vi "Programer.vi"(7 "ID":T1, 8 "error in":errorcluster, 9 "version path":path=path "C:/4.9.12.6034", 10 "Boolean refs":refnum<vi>[](array[refnum]), 11 "Commands":string[](array[string])) -> (0 "error out":errorcluster, 1 "error?":bool, 2 "Checksum":string, 3 "Response":string)   [LabVIEW 2021]
uses:
  controls/ID.ctl
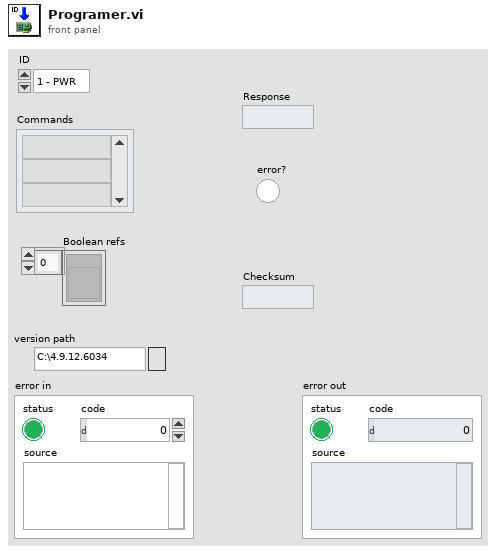
[diagram p1: front panel]
types:
  T1 = typedef "ID.ctl" = enum16{"1 - PWR", "2 - SM", "3 - DC", "4 - DM", "5 - WS", "6 - DS", "7 - WC", "8 - WA", "9 - WM", "10 - DA", "11 - WH", "12 - DH"}
  T2 = cluster{"accent s color":u32, "accent s color":u32}
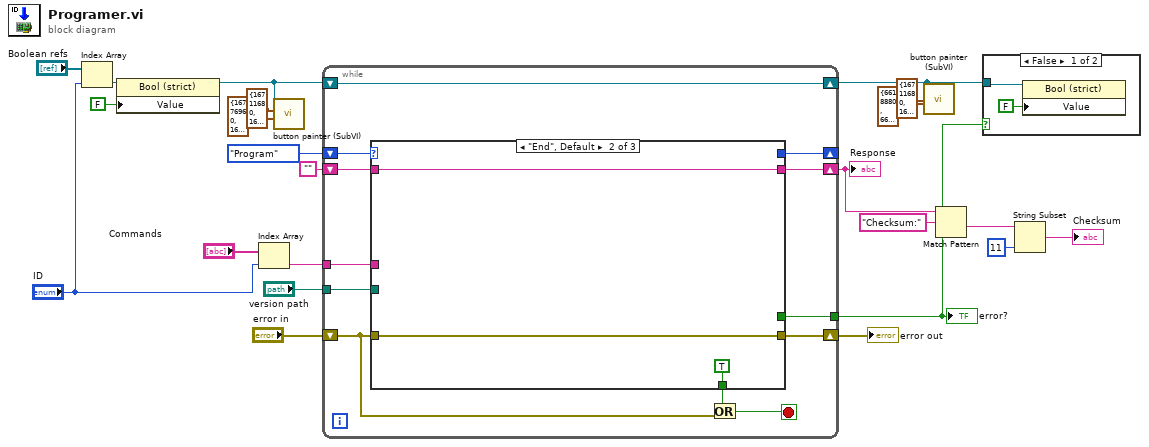
[diagram p0: block diagram]
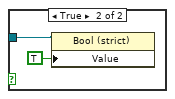
[diagram p2: hidden frame]
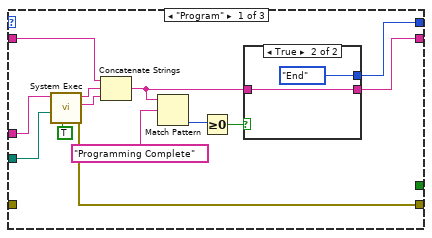
[diagram p3: hidden frame]
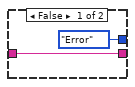
[diagram p4: hidden frame]
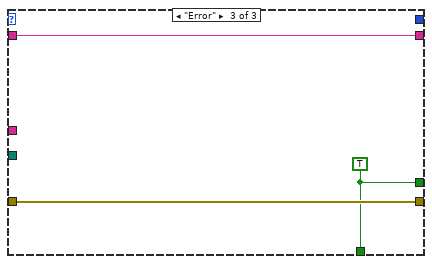
[diagram p5: hidden frame]
diagram:
  n1 = Index Array(array="Boolean refs", index="ID") -> (element=w7:refnum<vi>)
  n2 = property class="Bool (strict)"(reference=w7, "Value"=FALSE) -> (reference out=w6:refnum<vi>)  [unwired: 1 in, 1 out]
  n3 = Index Array(array="Commands", index="ID") -> (element=w22:string)
  n4 = call "button painter (SubVI).vi"("Off state"=cluster{"accent color":u32, "accent color":u32} {"accent color"=16776960, "accent color"=16776960}, "On state"=T2 {"accent s color"=16711680, "accent s color"=16711680}, "Button ref in"=w6) -> ()  [unwired: 9 in]
  n5 = while {
    shift-right: [w24] -> _
    shift-left: enum16{"Program", "End", "Error"}."Program" -> [w25]
    shift-right: [w35] -> w2
    shift-left: "" -> [w33]
    tunnel: w22 -> [w34]
    tunnel: [w32] -> w12
    shift-right: [w28] -> w20
    shift-left: "error in" -> [w29]
    tunnel: "version path" -> [w27]
    shift-right: [w26] -> w13
    shift-left: w6 -> [w26]
    stop <- w31 stop-if-true
    n6 = case shown="\"End\", Default" w25 {
      tunnel: [w40 w54 w58] -> w35
      tunnel: w34 -> [w42 _ _]
      tunnel: w33 -> [w41 w54 w58]
      tunnel: [_ TRUE w56] -> w30
      tunnel: [_ _ w56] -> w32
      tunnel: w29 -> [_ w55 w57]
      tunnel: [w39 w55 w57] -> w28
      tunnel: w27 -> [w38 _ _]
      tunnel: [w36 _ _] -> w24
      frame "Program" {
        n7 = call <vilib>:"System Exec.vi"("run minimized? (F)"=TRUE, "working directory"=w38, "command line"=w42) -> ("error out"=w39:errorcluster, "standard error"=w47:string, "standard output"=w48:string)  [unwired: 5 in, 1 out]
        n8 = Concatenate Strings(w41, w48, w47) -> (w43:string)
        n9 = Match Pattern(string=w43, regular expression="Programming Complete") -> (offset past match=w46:i32)  [unwired: 1 in, 3 out]
        n10 = Greater Or Equal To 0?(x=w46) -> (x >= 0?=w44:bool)
        n11 = case shown="True" w44 {
          tunnel: w43 -> [w50 w52]
          tunnel: [w50 w52] -> w40
          tunnel: [enum16{"Program", "End", "Error"}."Error" enum16{"Program", "End", "Error"}."End"] -> w36
          frame False {
          }
          frame True {
          }
        }
      }
      frame "End", Default {
      }
      frame "Error" {
        w56 = TRUE
      }
    }
    n12 = Or(x=w30, y=w29) -> (x .or. y?=w31:bool)
  }
  "error?" <- w12
  "error out" <- w20
  "Response" <- w2
  n13 = call "button painter (SubVI).vi"("Off state"=cluster{"accent color":u32, "accent color":u32} {"accent color"=6618880, "accent color"=6618880}, "On state"=T2 {"accent s color"=16711680, "accent s color"=16711680}, "Button ref in"=w13) -> ()  [unwired: 9 in]
  n14 = Match Pattern(string=w2, regular expression="Checksum:") -> (after substring=w4:string)  [unwired: 1 in, 3 out]
  n15 = case shown="False" w12 {
    tunnel: w13 -> [w59 w62]
    frame False {
      n16 = property class="Bool (strict)"(reference=w59, "Value"=FALSE) -> ()  [unwired: 1 in, 2 out]
    }
    frame True {
      n17 = property class="Bool (strict)"(reference=w62, "Value"=TRUE) -> ()  [unwired: 1 in, 2 out]
    }
  }
  n18 = String Subset(string=w4, length (rest)=11 ("length (rest)")) -> (substring=→"Checksum":string)  [unwired: 1 in]
